vi "Inspect.vi"(8 "Error in":errorcluster, 9 "Msg":refnum<class "Msg.lvclass">, 10 "Within Unified Msgs":bool, 11 "Base Actor in":refnum<class "Base Actor.lvclass">) -> (2 "Proceed":bool=TRUE, 3 "Base Actor out":refnum<class "Base Actor.lvclass">)   [LabVIEW 2025, in "jettl.lvlib" / "Base jettl Actor.lvlib" / "Base Actor.lvlib" / "Base Actor.lvclass"]
uses:
  Base Actor.lvclass
  Msg/Msg.lvclass
  Base Actor.lvclass/Base Actor.ctl
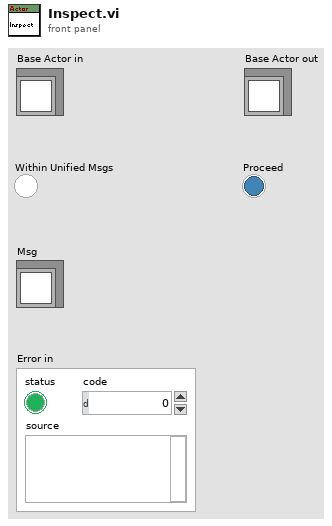
[diagram p1: front panel]
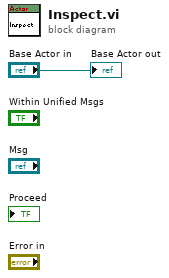
[diagram p0: block diagram]
diagram:
  "Base Actor out" <- "Base Actor in"
